vi "destroy this.vi"(0 "i ref in":refnum<vi>, 2 "unload process":bool, 3 "close FP first":bool, 4 "CallType":enum16{"simple", "synchronous", "asynchronous"}(ring)) -> (17 "obj destroyed":bool)   [LabVIEW 2014, in "PTUtils.lvlib"]
uses:
  PTUtils.lvlib
  CS_Core/CSSystem/CoreLib/CoreLib.string 2 byte array.vi
  CS_Core/CSSystem/CSSystemLib/CSSystemLib.lvlib
  CS_Core/CSSystem/CoreLib/CoreLib.lvlib
  CS_Core/CSSystem/CSAccessLib/CSAccessLib.lvlib
  CS_Core/CSObj/CSObj.lvlib
  CS_Core/BaseProcess/BaseProcess.lvlib
panel:
  in  "Case Constant\n(See Context Help)":bool
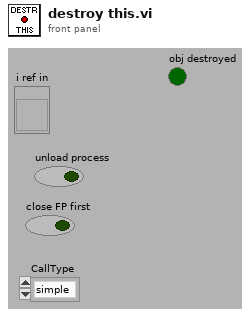
[diagram p1: front panel]
types:
  T1 = typedef "CoreDefs.rawDataType.ctl" = i8[]
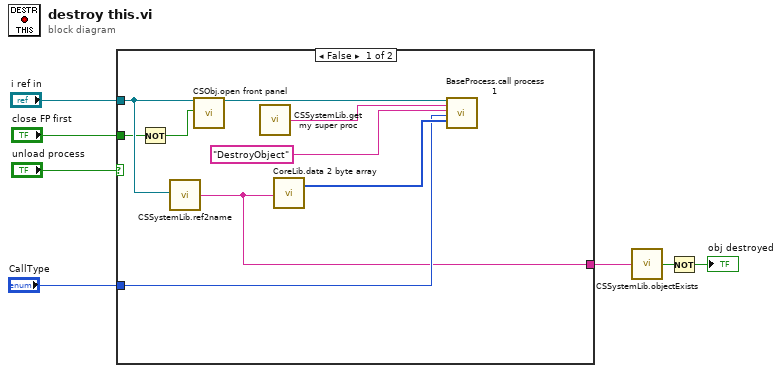
[diagram p0: block diagram]
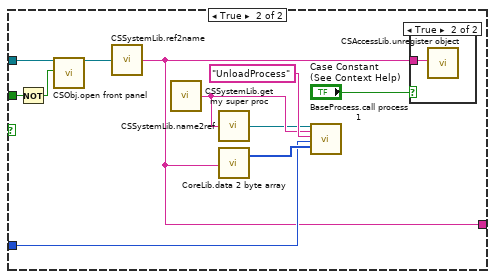
[diagram p2: hidden frame]
diagram:
  n1 = case shown="False" "unload process" {
    tunnel: "i ref in" -> [w13 w19]
    tunnel: "close FP first" -> [w11 w20]
    tunnel: "CallType" -> [w9 w22]
    tunnel: [w8 w17] -> w3
    frame False {
      n2 = Not(x=w11) -> (.not. x?=w10:bool)
      n3 = call "CSSystemLib.ref2name.vi"("obj refnum"=w13) -> ("name"=w8:string)
      n4 = call "CSObj.open front panel.vi"("i ref in"=w13, "frontPanelOpen"=w10) -> ("i ref out"=w12:refnum<vi>)  [unwired: 16 in, 1 out]
      n5 = call "CSSystemLib.get my super proc.vi"() -> ("name"=w15:string)  [unwired: 1 in]
      n6 = call-poly "CoreLib.data 2 byte array.vi"("string"=w8) -> ("byteArray out"=w16:T1)  [unwired: 18 in]
      n7 = call "BaseProcess.call process 1.vi"("i ref in"=w12, "Object"=w15, "Selector"="DestroyObject", "CallType"=w9, "Data"=w16) -> ()  [unwired: 12 in, 3 out]
    }
    frame True {
      n8 = Not(x=w20) -> (.not. x?=w21:bool)
      n9 = call "CSObj.open front panel.vi"("i ref in"=w19, "frontPanelOpen"=w21) -> ("i ref out"=w18:refnum<vi>)  [unwired: 16 in, 1 out]
      n10 = call "CSSystemLib.ref2name.vi"("obj refnum"=w18) -> ("name"=w17:string)
      n11 = call "CSSystemLib.get my super proc.vi"() -> ("name"=w24:string)  [unwired: 1 in]
      n12 = call "CSSystemLib.name2ref.vi"("name"=w24) -> ("obj refnum"=w23:refnum<vi>)
      n13 = call-poly "CoreLib.data 2 byte array.vi"("string"=w17) -> ("byteArray out"=w27:T1)  [unwired: 18 in]
      n14 = call "BaseProcess.call process 1.vi"("i ref in"=w23, "Object"=w24, "Selector"="UnloadProcess", "CallType"=w22, "Data"=w27) -> ()  [unwired: 12 in, 3 out]
      n15 = case shown="True" "Case Constant\n(See Context Help)" {
        tunnel: w17 -> [_ w28]
        frame False {
        }
        frame True {
          n16 = call "CSAccessLib.unregister object.vi"("objectName"=w28) -> ()  [unwired: 18 in, 1 out]
        }
      }
    }
  }
  n17 = call "CSSystemLib.objectExists.vi"("name"=w3) -> ("obj exists"=w2:bool)
  n18 = Not(x=w2) -> (.not. x?=→"obj destroyed":bool)
